vi "Page_Info_Validate_Filename.vi"(8 "error in (no error)":errorcluster, 10 "Filename in":string, 11 "AB_Targetfile in":refnum<class "AB_Targetfile.lvclass">) -> (0 "error out":errorcluster, 1 "hasInvalidCharacters":bool, 2 "Filename out":string, 3 "AB_Targetfile out":refnum<class "AB_Targetfile.lvclass">, 5 "message":string)   [LabVIEW 2020, in "AB_Targetfile.lvclass"]
uses:
  <vilib>/AppBuilder/AB_Classes/TargetFile/AB_Targetfile.lvclass
  <resource>/Framework/Providers/Common/provcom_StringGlobals.vi
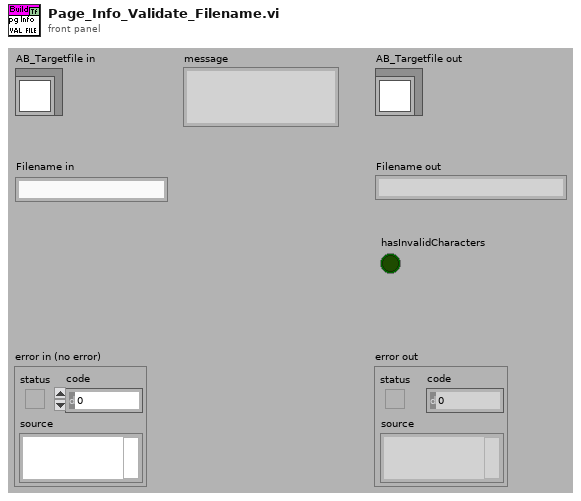
[diagram p1: front panel]
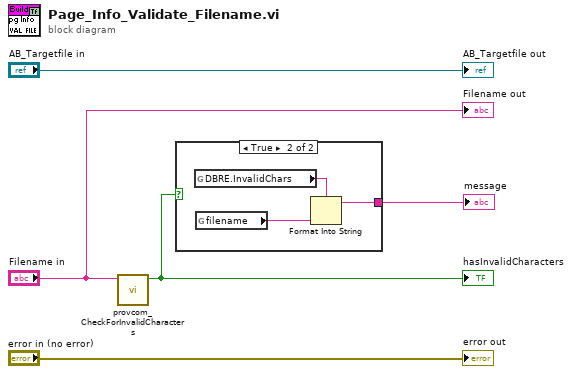
[diagram p0: block diagram]
diagram:
  n1 = call <resource>:"provcom_CheckForInvalidCharacters.vi"("NewString"="Filename in") -> ("HasInvalidCharacters"=w1:bool)  [unwired: 9 in, 1 out]
  "hasInvalidCharacters" <- w1
  n2 = case shown="True" w1 {
    tunnel: [_ w6] -> w2
    frame False {
    }
    frame True {
      n3 = global read "provcom_StringGlobals.vi" "DBRE.InvalidChars"() -> (w7:string)
      n4 = global read "provcom_StringGlobals.vi" "filename"() -> (w8:string)
      n5 = Format Into String(format string=w7, w8) -> (resulting string=w6:string)  [unwired: 2 in, 1 out]
    }
  }
  "message" <- w2
  "error out" <- "error in (no error)"
  "AB_Targetfile out" <- "AB_Targetfile in"
  "Filename out" <- "Filename in"
